vi "ProjetAsservissementTemperature.vi"() -> ()   [LabVIEW 2021]
doc: "Le protocole UDP diffère du protocole TCP car il n'y a pas de détection d'erreur avec les paquets d'informations qui sont envoyés ; il n'y a donc aucune garantie qu'un destinataire reçoive bien des données.\n\nLe protocole UDP offre la possibilité de diffuser des données sur un réseau. Spécifiez simplement une adresse IP de uns (255.255.255.255) pour essayer de diffuser l'information sur tout le réseau. Gardez à l'esprit que des routeurs et d'autres périphériques de réseau refusent généralement de diffuser au-delà de certains points, la diffusion est donc limitée dans la pratique."
panel:
  in  "Période (en ms)":u32=1000 min=500 max=10000 step=500
  out "(sup.inf)":u16
  out "entier 16 bits non signé":u16[](array[numeric])
  out "*(type *) &x":string
  out "sous-tableau":u8[](array[numeric])
  out "Graphe déroulant":dbl(graph)
  out "Cmd [ V | F | A0 | A1 ] 2":i8[](array[numeric])
  in  "Instruction\n[1] Get Analog\n[2] Set Digital (PWM)":u8=1 min=1 max=2
  out "Réponse":u8[](array[numeric])
  in  "Arrêter":bool
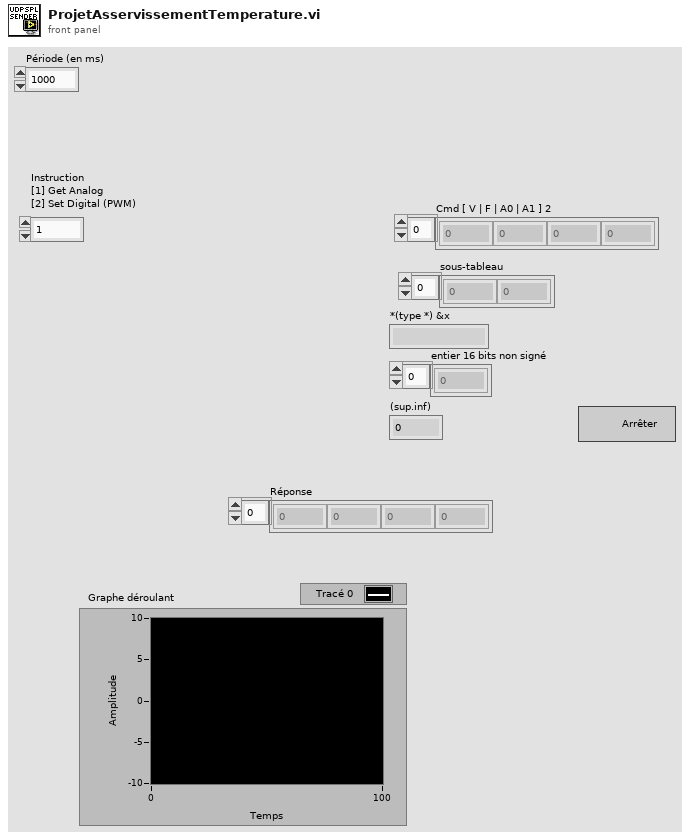
[diagram p1: front panel]
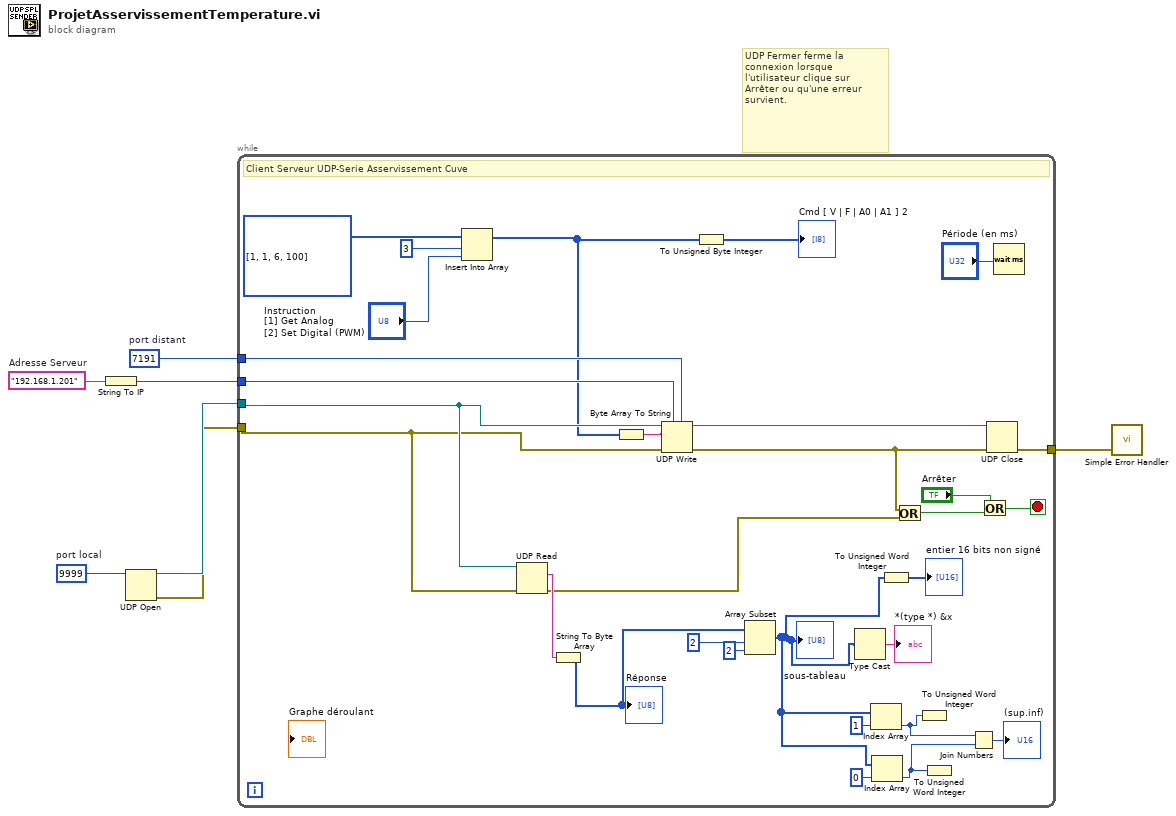
[diagram p0: block diagram]
diagram:
  w2 = u16 7191  # port distant
  w3 = u16 9999  # port local
  w7 = "192.168.1.201"  # Adresse Serveur
  # "UDP Fermer ferme la connexion lorsque l'utilisateur clique sur Arrêter ou qu'une erreur survient."
  n1 = String To IP(1:w7) -> (0:w6:u32)
  n2 = UDP Open(11:w3) -> (port=w5:refnum<k16>, 0:w4:errorcluster)  [unwired: 4 in, 1 out]
  n3 = while {
    tunnel: w5 -> [w34]
    tunnel: w4 -> [w17]
    tunnel: w6 -> [w37]
    tunnel: w2 -> [w36]
    tunnel: [w15] -> w1
    stop <- w10 stop-if-true
    # "Client Serveur UDP-Serie Asservissement Cuve"
    n4 = Insert Into Array(array=i32[] [1, 1, 6, 100], index=3 ("indice"), new element="Instruction\n[1] Get Analog\n[2] Set Digital (PWM)") -> (w29:i32[])
    n5 = UDP Read(connection ID=w34, 8:w17) -> (data out=w33:string, error out=w14:errorcluster)  [unwired: 2 in, 3 out]
    n6 = String To Byte Array(string=w33) -> (unsigned byte array=w28:u8[])
    "Réponse" <- w28
    n7 = Byte Array To String(unsigned byte array=w29) -> (string=w35:string)
    n8 = UDP Write(address=w37, port or service name=w36, connection ID=w34, data in=w35, 8:w17) -> (error out=w13:errorcluster, 3:w16:refnum<k16>)  [unwired: 1 in]
    n9 = To Unsigned Byte Integer(number=w29) -> (unsigned 8bit integer=→"Cmd [ V | F | A0 | A1 ] 2":u8[])
    n10 = Array Subset(array=w28, index=2 ("indice"), length=2 ("longueur")) -> (w21:u8[])
    "sous-tableau" <- w21
    n11 = Type Cast(x=w21) -> (*(type *) &x=→"*(type *) &x":string)  [unwired: 1 in]
    n12 = Index Array(array=w21, index=1 ("indice")) -> (element=w20:u8)
    n13 = Index Array(array=w21, index=0 ("indice")) -> (element=w19:u8)
    n14 = To Unsigned Word Integer(number=w21) -> (unsigned 16bit integer=→"entier 16 bits non signé":u16[])
    n15 = Or(x=w13, y=w14) -> (x .or. y?=w12:bool)
    n16 = To Unsigned Word Integer(number=w20) -> ()  [unwired: 1 out]
    n17 = To Unsigned Word Integer(number=w19) -> ()  [unwired: 1 out]
    n18 = Join Numbers(hi=w20, lo=w19) -> ((hi.lo)=→"(sup.inf)":u16)
    n19 = Or(x="Arrêter", y=w12) -> (x .or. y?=w10:bool)
    n20 = UDP Close(connection ID=w16, 8:w13) -> (error out=w15:errorcluster)  [unwired: 1 out]
    n21 = Wait (ms)(milliseconds to wait="Période (en ms)") -> ()  [unwired: 1 out]
  }
  n22 = call <vilib>:"Simple Error Handler.vi"("error in (no error)"=w1) -> ()  [unwired: 4 in, 5 out]
